vi "Obtain Request Events.vi"(8 "error in (no error)":errorcluster, 10 "Create New? (F)":bool) -> (0 "error out":errorcluster, 2 "ExampleClone Request Events":T1)   [LabVIEW 2022 SP3, in "ExampleClone.lvlib"]
doc: "This VI Obtains/Creates the Requests events that will be used for other modules to communicate with the module that owns this VI. These Requests events will be accessed only via Public API methods for this module.\n\n<b>NOTE</b>: The contents of this VI are automatically generated and modified by the <b>Tools > Delacor > DQMH</b> utilities. Consider using those utilities instead of making your own modifications to this VI.\n____\nHAMPEL SOFTWARE ENGINEERING v2.6.0 (2023-12-19 10:54)"
uses:
  ExampleClone.lvlib
  Request Events--cluster.ctl
  Stop Argument--cluster.ctl
  Show Panel Argument--cluster.ctl
  Hide Panel Argument--cluster.ctl
  Show Diagram Argument--cluster.ctl
  Get Module Execution Status Argument--cluster.ctl
  Request UI Display Argument--cluster.ctl
  Libraries/hse-libraries/Source/hse-dqmh/Controls/Module Display Scenarios.ctl
  Request UI Display (Reply Payload)--cluster.ctl
  Configure Argument--cluster.ctl
  Prepare Argument--cluster.ctl
  ExampleMessage Argument--cluster.ctl
  Libraries/hse-libraries/Source/hse-dqmh/hse-dqmh.lvlib
panel:
  # "NOTE: The contents of this VI are automatically generated and modified by the Tools > Delacor > DQMH utilities. Consider using those utilities instead of making your own modifications to this VI."
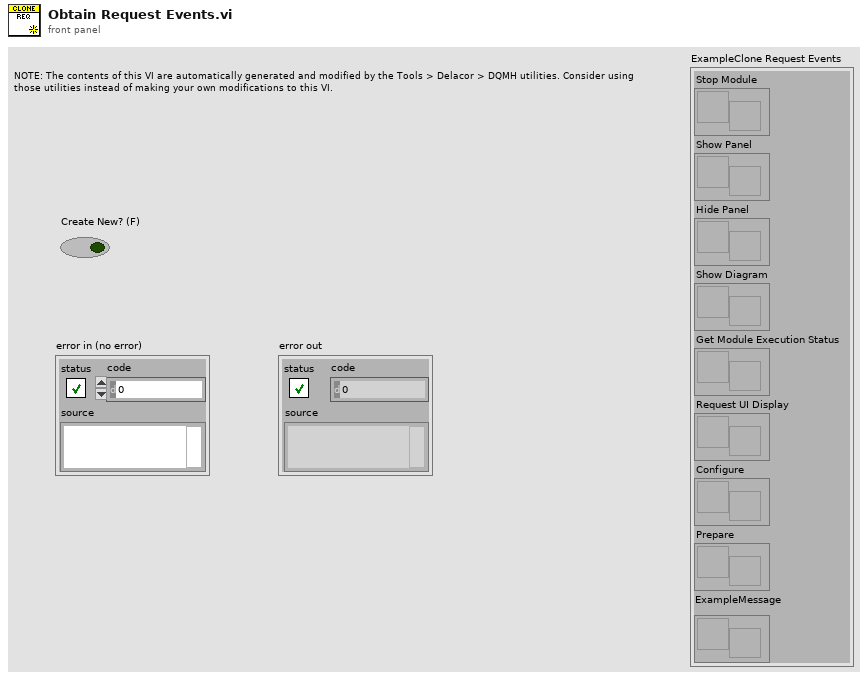
[diagram p1: front panel]
types:
  T1 = typedef "ExampleClone.lvlib/Request Events--cluster.ctl" = cluster{"Stop Module":refnum<user-event>, "Show Panel":refnum<user-event>, "Hide Panel":refnum<user-event>, "Show Diagram":refnum<user-event>, "Get Module Execution Status":refnum<user-event>, "Request UI Display":refnum<user-event>, "Configure":refnum<user-event>, "Prepare":refnum<user-event>, "ExampleMessage":refnum<user-event>}
  T2 = typedef "ExampleClone.lvlib/ExampleMessage Argument--cluster.ctl" = cluster{"Module ID":i32, "ExampleMessage":string}
  T3 = typedef "ExampleClone.lvlib/Prepare Argument--cluster.ctl" = cluster{"Module ID":i32, "Boolean":bool}
  T4 = typedef "ExampleClone.lvlib/Configure Argument--cluster.ctl" = cluster{"Module ID":i32, "Boolean":bool}
  T5 = typedef "ExampleClone.lvlib/Request UI Display Argument--cluster.ctl" = cluster{"Module ID":i32, "Scenario":T6, "Wait Notifier":refnum<notifier>, "wait for reply":bool}
  T6 = typedef "hse-dqmh.lvlib/Module Display Scenarios.ctl" = enum16{"Stand-Alone", "Managed"}
  T7 = typedef "ExampleClone.lvlib/Get Module Execution Status Argument--cluster.ctl" = cluster{"Module ID":i32, "Running?":bool}
  T8 = typedef "ExampleClone.lvlib/Show Diagram Argument--cluster.ctl" = cluster{"Module ID":i32, "Debug?":bool}
  T9 = typedef "ExampleClone.lvlib/Show Panel Argument--cluster.ctl" = cluster{"Module ID":i32, "Show Panel?":bool}
  T10 = typedef "ExampleClone.lvlib/Hide Panel Argument--cluster.ctl" = cluster{"Module ID":i32, "Hide Panel?":bool}
  T11 = typedef "ExampleClone.lvlib/Stop Argument--cluster.ctl" = cluster{"Module ID":i32, "Origin":string, "Exit via Stop Module Req?":bool, "Wait for Module to stop?":bool}
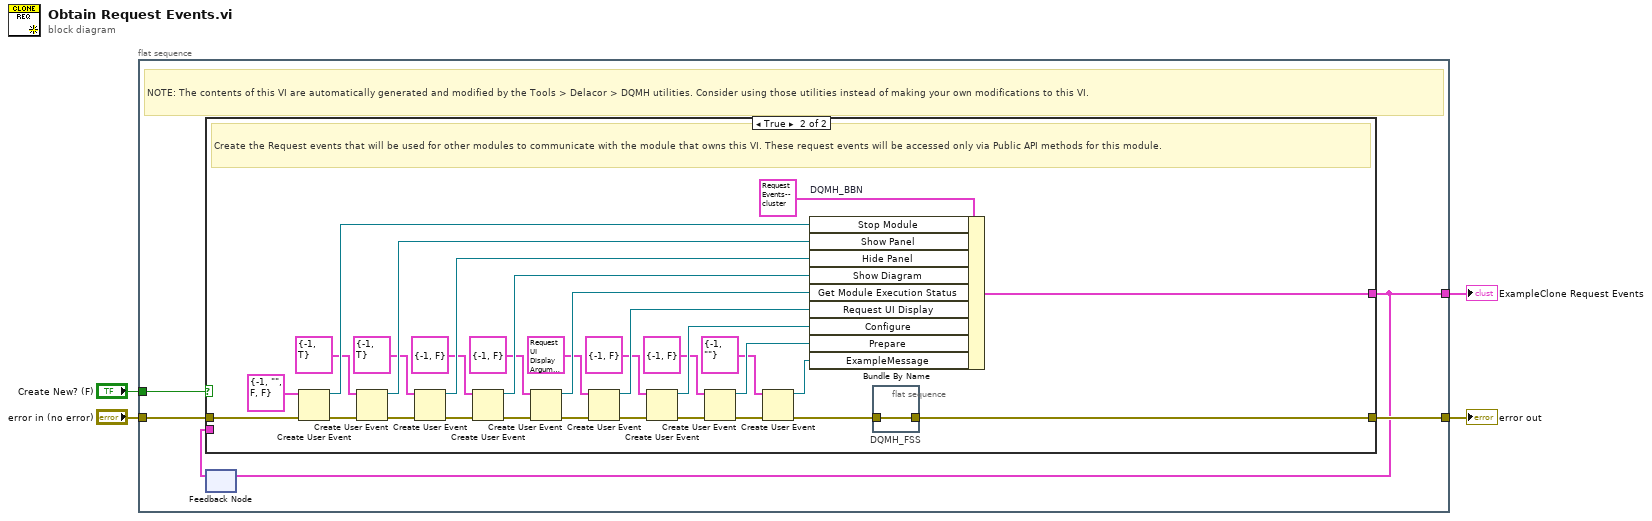
[diagram p0: block diagram]
diagram:
  n1 = flat-sequence {
    tunnel: [w9] -> w4
    tunnel: "error in (no error)" -> [w8]
    tunnel: [w6] -> w2
    tunnel: "Create New? (F)" -> [w5]
    frame #0 {
      # "NOTE: The contents of this VI are automatically generated and modified by the Tools > Delacor > DQMH utilities. Consider using those utilities instead of making your own modifications to this VI."
      n2 = feedback #1() -> (w7:T1)  [unwired: 1 in]
      n3 = case shown="True" w5 {
        tunnel: [w10 w30] -> w9
        tunnel: w8 -> [w10 w42]
        tunnel: [w11 w39] -> w6
        tunnel: w7 -> [w11 _]
        frame False {
        }
        frame True {
          # "Create the Request events that will be used for other modules to communicate with the module that owns this VI. These request events will be accessed only via Public API methods for this module."
          n4 = Create User Event(user event datatype=T11 {"Module ID"=-1, "Origin"="", "Exit via Stop Module Req?"=FALSE, "Wait for Module to stop?"=FALSE} ("Stop Argument"), error in=w42) -> (user event=w40:refnum<user-event>, error out=w37:errorcluster)
          n5 = Create User Event(user event datatype=T9 {"Module ID"=-1, "Show Panel?"=TRUE} ("Show Panel Argument"), error in=w37) -> (user event=w36:refnum<user-event>, error out=w34:errorcluster)
          n6 = Create User Event(user event datatype=T10 {"Module ID"=-1, "Hide Panel?"=TRUE} ("Hide Panel"), error in=w34) -> (user event=w33:refnum<user-event>, error out=w32:errorcluster)
          n7 = Create User Event(user event datatype=T8 {"Module ID"=-1, "Debug?"=FALSE} ("Show Diagram Argument"), error in=w32) -> (user event=w28:refnum<user-event>, error out=w29:errorcluster)
          n8 = Create User Event(user event datatype=T7 {"Module ID"=-1, "Running?"=FALSE} ("Get Module Execution Status Argument"), error in=w29) -> (user event=w25:refnum<user-event>, error out=w26:errorcluster)
          n9 = Create User Event(user event datatype=T5 {"Module ID"=-1, "Scenario"=enum."Stand-Alone", "Wait Notifier"=refnum, "wait for reply"=FALSE} ("Request UI Display Argument"), error in=w26) -> (user event=w22:refnum<user-event>, error out=w23:errorcluster)
          n10 = Create User Event(user event datatype=T4 {"Module ID"=-1, "Boolean"=FALSE} ("Configure Argument"), error in=w23) -> (user event=w19:refnum<user-event>, error out=w20:errorcluster)
          n11 = Create User Event(user event datatype=T3 {"Module ID"=-1, "Boolean"=FALSE} ("Prepare Argument"), error in=w20) -> (user event=w16:refnum<user-event>, error out=w17:errorcluster)
          n12 = Create User Event(user event datatype=T2 {"Module ID"=-1, "ExampleMessage"=""} ("ExampleMessage Argument"), error in=w17) -> (user event=w13:refnum<user-event>, error out=w14:errorcluster)
          n13 = Bundle By Name "DQMH_BBN"(cluster=T1 {"Stop Module"=refnum, "Show Panel"=refnum, "Hide Panel"=refnum, "Show Diagram"=refnum, "Get Module Execution Status"=refnum, "Request UI Display"=refnum, "Configure"=refnum, "Prepare"=refnum, "ExampleMessage"=refnum} ("output cluster"), "Stop Module"=w40, "Show Panel"=w36, "Hide Panel"=w33, "Show Diagram"=w28, "Get Module Execution Status"=w25, "Request UI Display"=w22, "Configure"=w19, "Prepare"=w16, "ExampleMessage"=w13) -> (w39:T1)
          n14 = flat-sequence "DQMH_FSS" {
            tunnel: w14 -> [w43]
            tunnel: [w43] -> w30
            frame #0 {
            }
          }
        }
      }
      n15 = feedback-in #1(w6) -> ()
    }
  }
  "ExampleClone Request Events" <- w2
  "error out" <- w4
